vi "CSMLS - Remove Loop Tag and previous State(s) to Break.vi"(11 "States Queue":string) -> (3 "Remaining States":string)   [LabVIEW 2017, in "CSM Loop Support.lvlib"]
doc: "Stops the loop by removing the `<loop>` tag and all states before the `<loop>` tag.\n\n<b>Example</b>: If the following messages exist in the CSM message queue, executing the current API operation will remove the messages where the comments are located.\n\n DAQ: Acquire // Will be removed\n DAQ: Continuous Check -><loop> // Will be removed\n DAQ: Stop\n DAQ: Close\n\nThis is equivalent to not executing any DAQ operations and immediately entering stop and release.\n\n-- <b>Controls</b> --\n- <b>States Queue</b>: Connect the entire state queue to this input.\n\n-- <b>Indicators</b> --\n- <b>Remaining States</b>: The remaining message queue."
uses:
  CSM Loop Support.lvlib
  Communicable State Machine.lvlib
  _Shared/CSM Shared.lvlib
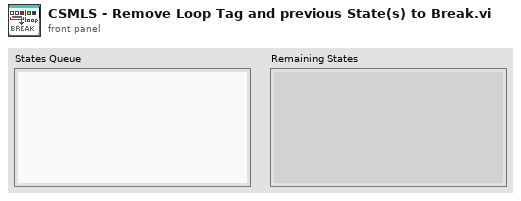
[diagram p1: front panel]
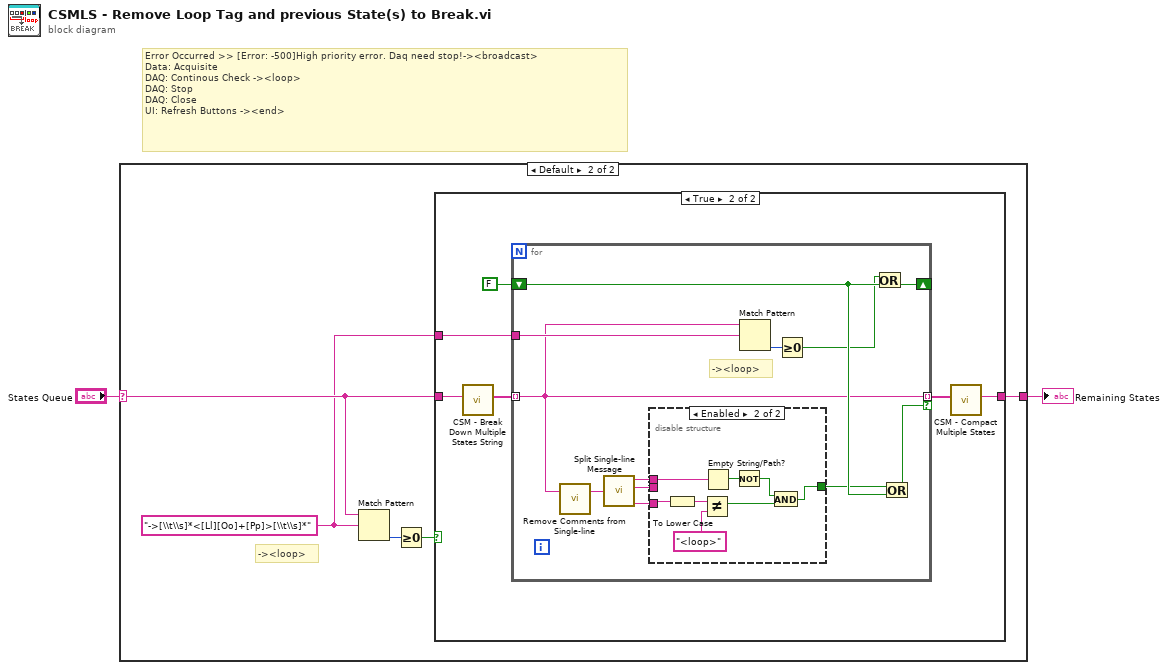
[diagram p0: block diagram]
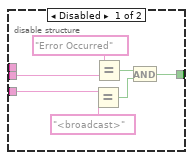
[diagram p4: hidden frame]
diagram:
  # "Error Occurred >> [Error: -500]High priority error. Daq need stop!-><broadcast>\nData: Acquisite\nDAQ: Continous Check -><loop>\nDAQ: Stop\nDAQ: Close\nUI: Refresh Buttons -><end>"
  n1 = case shown="Default" "States Queue" {
    selector: "States Queue" -> [w3 w6]
    tunnel: [w3 w8] -> w2
    frame "" {
    }
    frame Default {
      w4 = "->[\\t\\s]*<[Ll][Oo]+[Pp]>[\\t\\s]*" ("regular expression")
      # "-><loop>"
      n2 = Match Pattern(string=w6, regular expression=w4) -> (offset past match=w7:i32)  [unwired: 1 in, 3 out]
      n3 = Greater Or Equal To 0?(x=w7) -> (x >= 0?=w5:bool)
      n4 = case shown="True" w5 {
        tunnel: [w9 w15] -> w8
        tunnel: w6 -> [w9 w14]
        tunnel: w4 -> [_ w13]
        frame False {
        }
        frame True {
          n5 = call "CSM - Break Down Multiple States String.vi"("States"=w14) -> ("Multiple States"=w12:string[])  [unwired: 10 in]
          n6 = for {
            tunnel: [w17] -> w11 mode=indexing if=w20
            tunnel: w12 -> [w17] mode=indexing
            shift-right: [w25] -> _
            shift-left: FALSE -> [w26]
            tunnel: w13 -> [w18]
            # "-><loop>"
            n7 = call "Remove Comments from Single-line.vi"("single-line text"=w17) -> ("single-line text without comments"=w23:string)  [unwired: 2 in]
            n8 = call "Split Single-line Message.vi"("single-line text"=w23) -> ("operator"=w16:string, "state"=w22:string, "source/target"=w21:string)  [unwired: 6 in, 1 out]
            n9 = disable-structure shown="Enabled" {
              disable-tunnel: w22 -> [w33 _]
              disable-tunnel: w21 -> [w31 w40]
              disable-tunnel: [w28 w36] -> w19
              disable-tunnel: w16 -> [_ w42]
              frame Disabled {
                n10 = Equal?(x=w31, y="<broadcast>") -> (x = y?=w29:bool)
                n11 = Equal?(x="Error Occurred", y=w33) -> (x = y?=w32:bool)
                n12 = And(x=w32, y=w29) -> (x .and. y?=w28:bool)
              }
              frame Enabled {
                n13 = To Lower Case(string=w40) -> (all lower case string=w35:string)
                n14 = Not Equal?(x=w35, y="<loop>") -> (x != y?=w37:bool)
                n15 = Empty String/Path?(string/path=w42) -> (empty?=w41:bool)
                n16 = Not(x=w41) -> (.not. x?=w38:bool)
                n17 = And(x=w38, y=w37) -> (x .and. y?=w36:bool)
              }
            }
            n18 = Match Pattern(string=w17, regular expression=w18) -> (offset past match=w27:i32)  [unwired: 1 in, 3 out]
            n19 = Greater Or Equal To 0?(x=w27) -> (x >= 0?=w24:bool)
            n20 = Or(x=w24, y=w26) -> (x .or. y?=w25:bool)
            n21 = Or(x=w19, y=w26) -> (x .or. y?=w20:bool)
          }
          n22 = call "CSM - Compact Multiple States.vi"("Multiple States"=w11) -> ("States"=w15:string)  [unwired: 9 in]
        }
      }
    }
  }
  "Remaining States" <- w2
